vi "CreatePrivateEvents.vi"(8 "error in (no error)":errorcluster, 11 "Instrument":refnum<class "Instrument.lvclass">) -> (0 "error out":errorcluster, 3 "Instrument out":refnum<class "Instrument.lvclass">)   [LabVIEW 2019, in "Instrument.lvclass"]
doc: "---------------------------------------------------------------\nJKI State Machine Objects™\nhttp://jki.net/state-machine-objects/\nCopyright (C) 2005-2015, JKI <info@jki.net>\nALL RIGHTS RESERVEDJKI State Machine Objects (SMO) 1.0.0.4\nJKI - JKI\nCopyright (c) 2015, JKI"
uses:
  Instrument.lvclass
  Typedefs/PrivateEvents--Instrument.MessageToProcess.ctl
  <userlib>/LevyLab/RemoteControl/RemoteControl/Typedefs/Message--Cluster.ctl
  Typedefs/PrivateEvents--Instrument.DataToLog.ctl
  Typedefs/PrivateEvents--LogTime.ctl
  Instrument.lvclass/Instrument.ctl
  <vilib>/JKI/JKI SMO/SMO/SMO.lvclass
  <userlib>/LevyLab/RemoteControl/RemoteControl/RemoteControl.lvclass
panel:
  # "For instructions on how to use the JKI State Machine Objects, examples and video tutorials, visit:\nhttp://jki.net/state-machine-objects/\n\nJKI State Machine Objects™\nhttp://jki.net/state-machine-objects/\nCopyright (C) 2005-2015, JKI <info@jki.net>\nALL RIGHTS RESERVED"
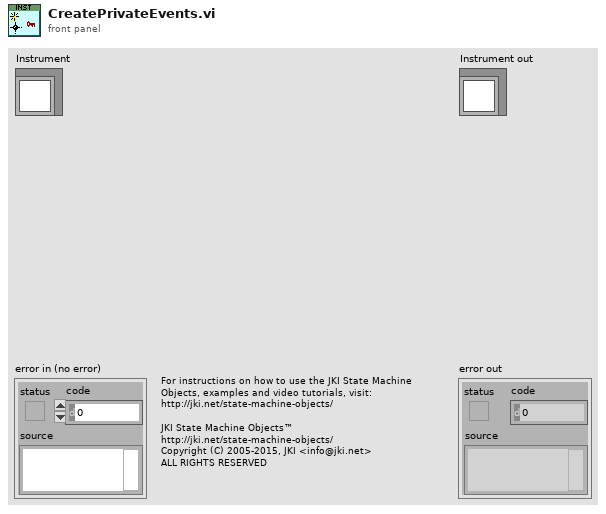
[diagram p1: front panel]
types:
  T1 = typedef "Instrument.lvclass/PrivateEvents--LogTime.ctl" = u32
  T2 = typedef "Instrument.lvclass/PrivateEvents--Instrument.DataToLog.ctl" = cluster{"Path(s)":string, "Data":variant}
  T3 = typedef "Instrument.lvclass/PrivateEvents--Instrument.MessageToProcess.ctl" = cluster{"Message":T4}
  T4 = typedef "RemoteControl.lvclass/Message--Cluster.ctl" = cluster{"Command":string, "Data":variant, "ID":string}
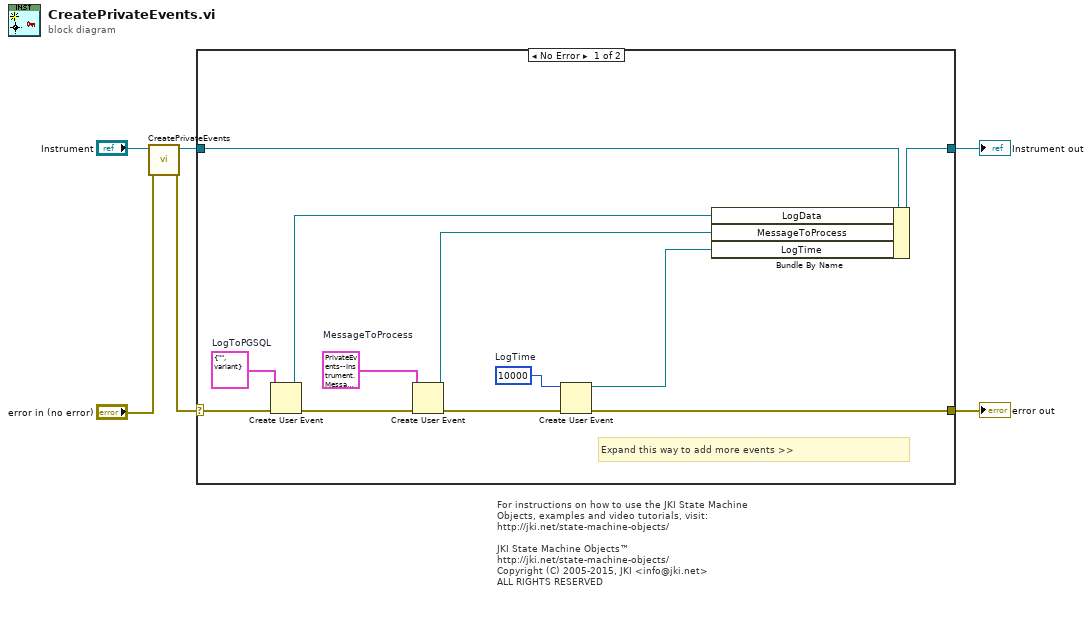
[diagram p0: block diagram]
diagram:
  # "For instructions on how to use the JKI State Machine Objects, examples and video tutorials, visit:\nhttp://jki.net/state-machine-objects/\n\nJKI State Machine Objects™\nhttp://jki.net/state-machine-objects/\nCopyright (C) 2005-2015, JKI <info@jki.net>\nALL RIGHTS RESERVED"
  n1 = call-parent "CreatePrivateEvents.vi"("error in (no error)"="error in (no error)", "SMO"="Instrument") -> ("error out"=w1:errorcluster, "SMO out"=w3:refnum<class "Instrument.lvclass">)  [unwired: 8 in]
  n2 = case shown="No Error" w1 {
    selector: w1 -> [w17 w20]
    tunnel: [w9 w20] -> w5
    tunnel: [w16 w19] -> w6
    tunnel: w3 -> [w18 w19]
    frame No Error {
      w8 = T1 10000  # LogTime
      w13 = T2 {"Path(s)"="", "Data"=variant(bool FALSE)}  # LogToPGSQL
      w15 = T3 {"Message"={"Command"="", "Data"=variant(string ""), "ID"=""}}  # MessageToProcess
      # "Expand this way to add more events >>"
      n3 = Create User Event(user event datatype=w13, error in=w17) -> (user event=w12:refnum<user-event>, error out=w14:errorcluster)
      n4 = Create User Event(user event datatype=w15, error in=w14) -> (user event=w11:refnum<user-event>, error out=w10:errorcluster)
      n5 = Create User Event(user event datatype=w8, error in=w10) -> (user event=w7:refnum<user-event>, error out=w9:errorcluster)
      n6 = Bundle By Name(cluster=w18, "LogData"=w12, "MessageToProcess"=w11, "LogTime"=w7) -> (w16:refnum<class "Instrument.lvclass">)
    }
    frame Error {
    }
  }
  "error out" <- w5
  "Instrument out" <- w6
